vi "Read TSP Net Remote Instrument Buffer Data.vi"(6 "Stop Index (2)":i32=2, 7 "Start Index (0)":i32, 8 "error in (no error)":errorcluster, 9 "Reading Buffer (smua.nvbuffer1)":string="smua.nvbuffer1", 10 "Instrument ID":string, 11 "VISA resource name":refnum<visa-resource-name>) -> (0 "error out":errorcluster, 2 "Buffer Data":dbl[](array[numeric]), 3 "VISA resource name out":refnum<visa-resource-name>)   [LabVIEW 2019, in "Keithley 2600 Series.lvlib"]
doc: "Returns a buffer synchronous table from a remote instrument, and copy it to to a TSP-enabled instrument. \n\n<b>Note:</b>\nThis VI only applies to the TSP-enabled instrument."
uses:
  Keithley 2600 Series.lvlib
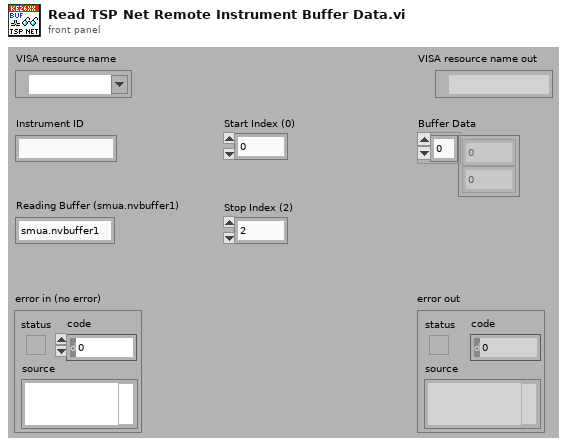
[diagram p1: front panel]
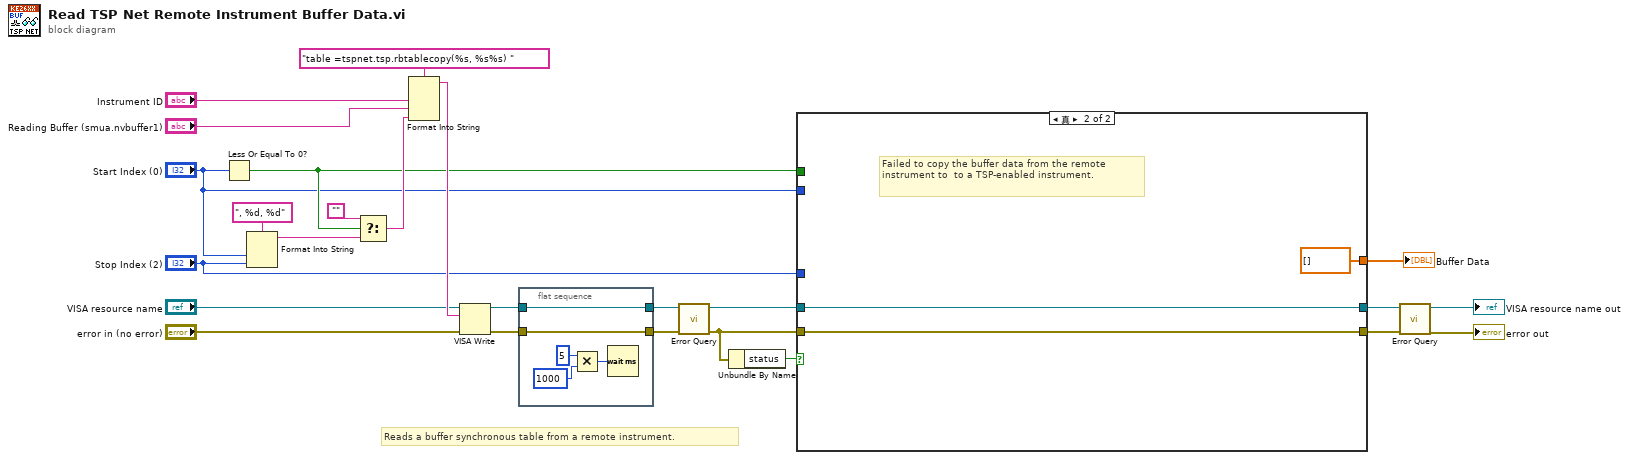
[diagram p0: block diagram]
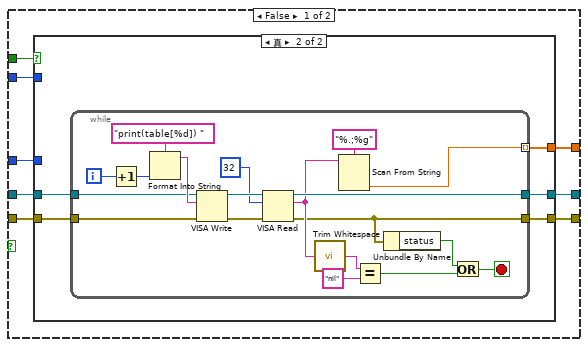
[diagram p2: hidden frame]
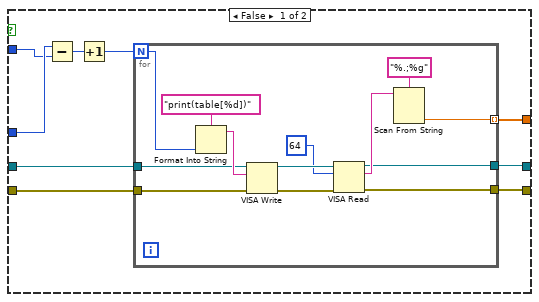
[diagram p3: hidden frame]
diagram:
  # "Reads a buffer synchronous table from a remote instrument."
  n1 = Less Or Equal To 0?(x="Start Index (0)") -> (x <= 0?=w14:bool)
  n2 = Format Into String(format string=", %d, %d", "Start Index (0)", "Stop Index (2)") -> (resulting string=w15:string)  [unwired: 2 in, 1 out]
  n3 = Select(t="", s=w14, f=w15) -> (s? t:f=w17:string)
  n4 = Format Into String(format string="table =tspnet.tsp.rbtablecopy(%s, %s%s) ", "Instrument ID", "Reading Buffer (smua.nvbuffer1)", w17) -> (resulting string=w22:string)  [unwired: 2 in, 1 out]
  n5 = VISA Write(VISA resource name="VISA resource name", write buffer=w22, error in (no error)="error in (no error)") -> (VISA resource name out=w10:refnum<visa-resource-name>, error out=w9:errorcluster)  [unwired: 1 out]
  n6 = flat-sequence {
    tunnel: w10 -> [w27]
    tunnel: w9 -> [w26]
    tunnel: [w27] -> w5
    tunnel: [w26] -> w4
    frame #0 {
      n7 = Multiply(x=5, y=1000) -> (x*y=w29:i32)
      n8 = Wait (ms)(milliseconds to wait=w29) -> ()  [unwired: 1 out]
    }
  }
  n9 = call "Error Query.vi"("error in (no error)"=w4, "VISA resource name"=w5) -> ("error out"=w2:errorcluster, "VISA resource name out"=w3:refnum<visa-resource-name>)  [unwired: 6 in, 2 out]
  n10 = Unbundle By Name(w2) -> ("status"=w1:bool)
  n11 = case shown="真" w1 {
    tunnel: w14 -> [w38 _]
    tunnel: "Start Index (0)" -> [w37 _]
    tunnel: "Stop Index (2)" -> [w36 _]
    tunnel: [w35 dbl[] []] -> w8
    tunnel: [w34 w86] -> w7
    tunnel: [w33 w87] -> w6
    tunnel: w3 -> [w32 w87]
    tunnel: w2 -> [w31 w86]
    frame False {
      n12 = case shown="真" w38 {
        tunnel: w32 -> [w40 w65]
        tunnel: w31 -> [w39 w64]
        tunnel: w37 -> [w46 _]
        tunnel: w36 -> [w47 _]
        tunnel: [w43 w62] -> w33
        tunnel: [w42 w61] -> w34
        tunnel: [w44 w63] -> w35
        frame False {
          n13 = Subtract(x=w47, y=w46) -> (x-y=w45:i32)
          n14 = Increment(x=w45) -> (x+1=w41:i32)
          n15 = for {
            N: w41 -> [w48]
            tunnel: [w60] -> w44 mode=indexing
            tunnel: w40 -> [w52]
            tunnel: w39 -> [w51]
            tunnel: [w50] -> w43
            tunnel: [w49] -> w42
            n16 = Format Into String(format string="print(table[%d])", w48) -> (resulting string=w56:string)  [unwired: 2 in, 1 out]
            n17 = VISA Write(VISA resource name=w52, write buffer=w56, error in (no error)=w51) -> (VISA resource name out=w59:refnum<visa-resource-name>, error out=w58:errorcluster)  [unwired: 1 out]
            n18 = VISA Read(VISA resource name=w59, byte count=u32 64, error in (no error)=w58) -> (VISA resource name out=w50:refnum<visa-resource-name>, read buffer=w54:string, error out=w49:errorcluster)  [unwired: 1 out]
            n19 = Scan From String(format string="%.;%g", input string=w54) -> (output 1=w60:dbl)  [unwired: 3 in, 3 out]
          }
        }
        frame True {
          n20 = while {
            tunnel: w65 -> [w75]
            tunnel: w64 -> [w74]
            tunnel: [w73] -> w62
            tunnel: [w69] -> w61
            tunnel: [w70] -> w63 mode=indexing
            i -> [w76]
            stop <- w68 stop-if-true
            n21 = Increment(x=w76) -> (x+1=w84:i32)
            n22 = Format Into String(format string="print(table[%d]) ", w84) -> (resulting string=w82:string)  [unwired: 2 in, 1 out]
            n23 = VISA Write(VISA resource name=w75, write buffer=w82, error in (no error)=w74) -> (VISA resource name out=w81:refnum<visa-resource-name>, error out=w80:errorcluster)  [unwired: 1 out]
            n24 = VISA Read(VISA resource name=w81, byte count=u32 32, error in (no error)=w80) -> (VISA resource name out=w73:refnum<visa-resource-name>, read buffer=w71:string, error out=w69:errorcluster)  [unwired: 1 out]
            n25 = call <vilib>:"Trim Whitespace.vi"("string"=w71) -> ("trimmed string"=w77:string)  [unwired: 1 in]
            n26 = Scan From String(format string="%.;%g", input string=w71) -> (output 1=w70:dbl)  [unwired: 3 in, 3 out]
            n27 = Equal?(x=w77, y="nil") -> (x = y?=w67:bool)
            n28 = Unbundle By Name(w69) -> ("status"=w66:bool)
            n29 = Or(x=w66, y=w67) -> (x .or. y?=w68:bool)
          }
        }
      }
    }
    frame True {
      # "Failed to copy the buffer data from the remote instrument to  to a TSP-enabled instrument."
    }
  }
  "Buffer Data" <- w8
  n30 = call "Error Query.vi"("error in (no error)"=w7, "VISA resource name"=w6) -> ("error out"=→"error out":errorcluster, "VISA resource name out"=→"VISA resource name out":refnum<visa-resource-name>)  [unwired: 6 in, 2 out]
